vi "ScanAction.vi"(8 "error in (no error)":errorcluster caption="entrée d'erreur (pas d'erreur)", 9 "IndicePoint":i32, 10 "Dir":bool, 11 "Device en entrée":refnum<class "BaseDevice.lvclass"> caption="DNL_LabVIEW Object in") -> (0 "error out":errorcluster caption="sortie d'erreur", 2 "ScanParsOut":dbl[](array[numeric]), 3 "Device en sortie":refnum<class "BaseDevice.lvclass"> caption="DNL_LabVIEW Object out")   [LabVIEW 2019, in "BaseDevice.lvclass"]
uses:
  BaseDevice.lvclass
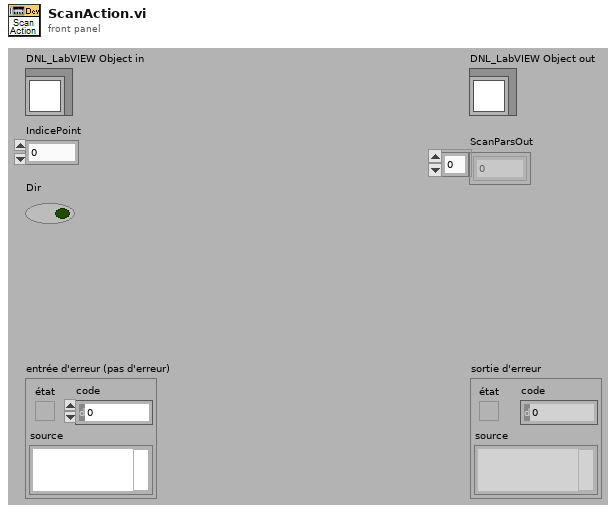
[diagram p1: front panel]
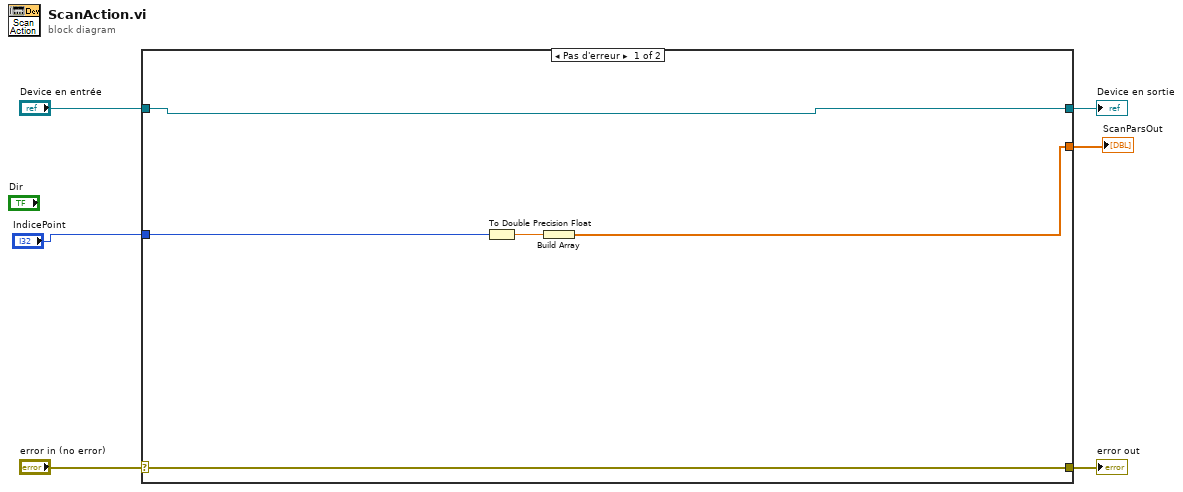
[diagram p0: block diagram]
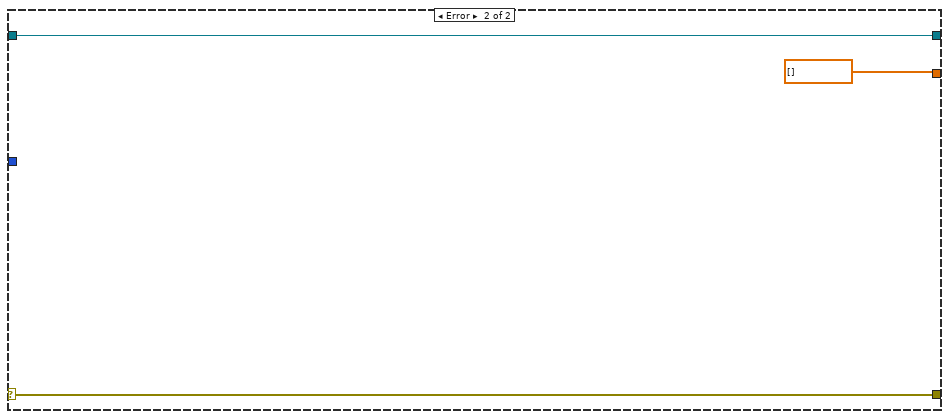
[diagram p2: hidden frame]
diagram:
  n1 = case shown="Pas d'erreur" "error in (no error)" {
    selector: "error in (no error)" -> [w10 w14]
    tunnel: [w10 w14] -> w5
    tunnel: [w11 w13] -> w3
    tunnel: "Device en entrée" -> [w11 w13]
    tunnel: [w7 dbl[] []] -> w2
    tunnel: "IndicePoint" -> [w9 _]
    frame No Error {
      n2 = To Double Precision Float(number=w9) -> (double precision float=w8:dbl)
      n3 = Build Array(w8) -> (w7:dbl[])
    }
    frame Error {
    }
  }
  "error out" <- w5
  "Device en sortie" <- w3
  "ScanParsOut" <- w2
